vi "Read Manifold Port.vi"(8 "error in":errorcluster, 10 "Manifold Port":i32, 11 "Gantry in":refnum<class "Gantry.lvclass">) -> (0 "error out":errorcluster, 2 "On/Off":bool, 3 "Gantry out":refnum<class "Gantry.lvclass">)   [LabVIEW 2024, in "Gantry.lvclass"]
uses:
  Gantry.lvclass
  FlexWorktable/FlexWorktable.lvclass
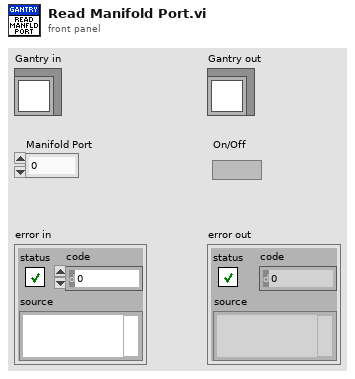
[diagram p1: front panel]
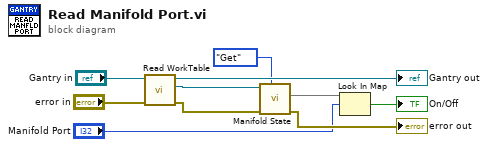
[diagram p0: block diagram]
diagram:
  n1 = call-dynamic "Read WorkTable.vi"("error in"="error in", "Gantry Class in"="Gantry in") -> ("error out"=w6:errorcluster, "Worktable"=w7:refnum<class "FlexWorktable.lvclass">, "Gantry Class out"=→"Gantry out":refnum<class "Gantry.lvclass">)  [unwired: 7 in]
  n2 = call-dynamic "Manifold State.vi"("Get/Set"=enum16{"Get", "Set"}."Get", "error in (no error)"=w6, "FlexWorktable in"=w7) -> ("error out"=→"error out":errorcluster, "Port Statuses"=w2:map{i32, bool})  [unwired: 6 in, 1 out]
  n3 = Look In Map(map=w2, key="Manifold Port") -> (key not found?=→"On/Off":bool)  [unwired: 1 in, 1 out]
